vi "MoveRelate.vi"(8 "error in (no error)":errorcluster, 11 "DMC 3600 in":refnum<class "DMC 3600.lvclass">) -> (0 "error out":errorcluster, 3 "DMC 3600 out":refnum<class "DMC 3600.lvclass">)   [LabVIEW 2019, in "DMC 3600.lvclass"]
uses:
  DMC 3600.lvclass
  LLB/Commonly VI.lvlib
  LLB/DMC3600/LTDMC.lvlib
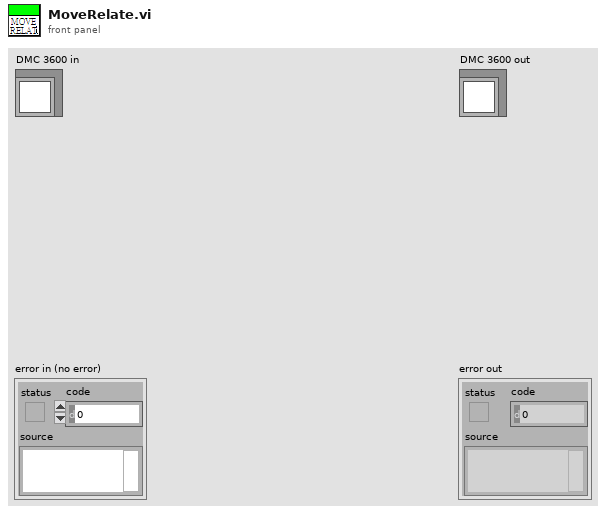
[diagram p1: front panel]
types:
  T1 = cluster{"AxisName":string, "Accel":dbl, "Deaccel":dbl, "Speed":dbl, "Sramp":dbl}[]
  T2 = cluster{"AxisName":string, "Accel":dbl, "Deaccel":dbl, "Speed":dbl, "Sramp":dbl}
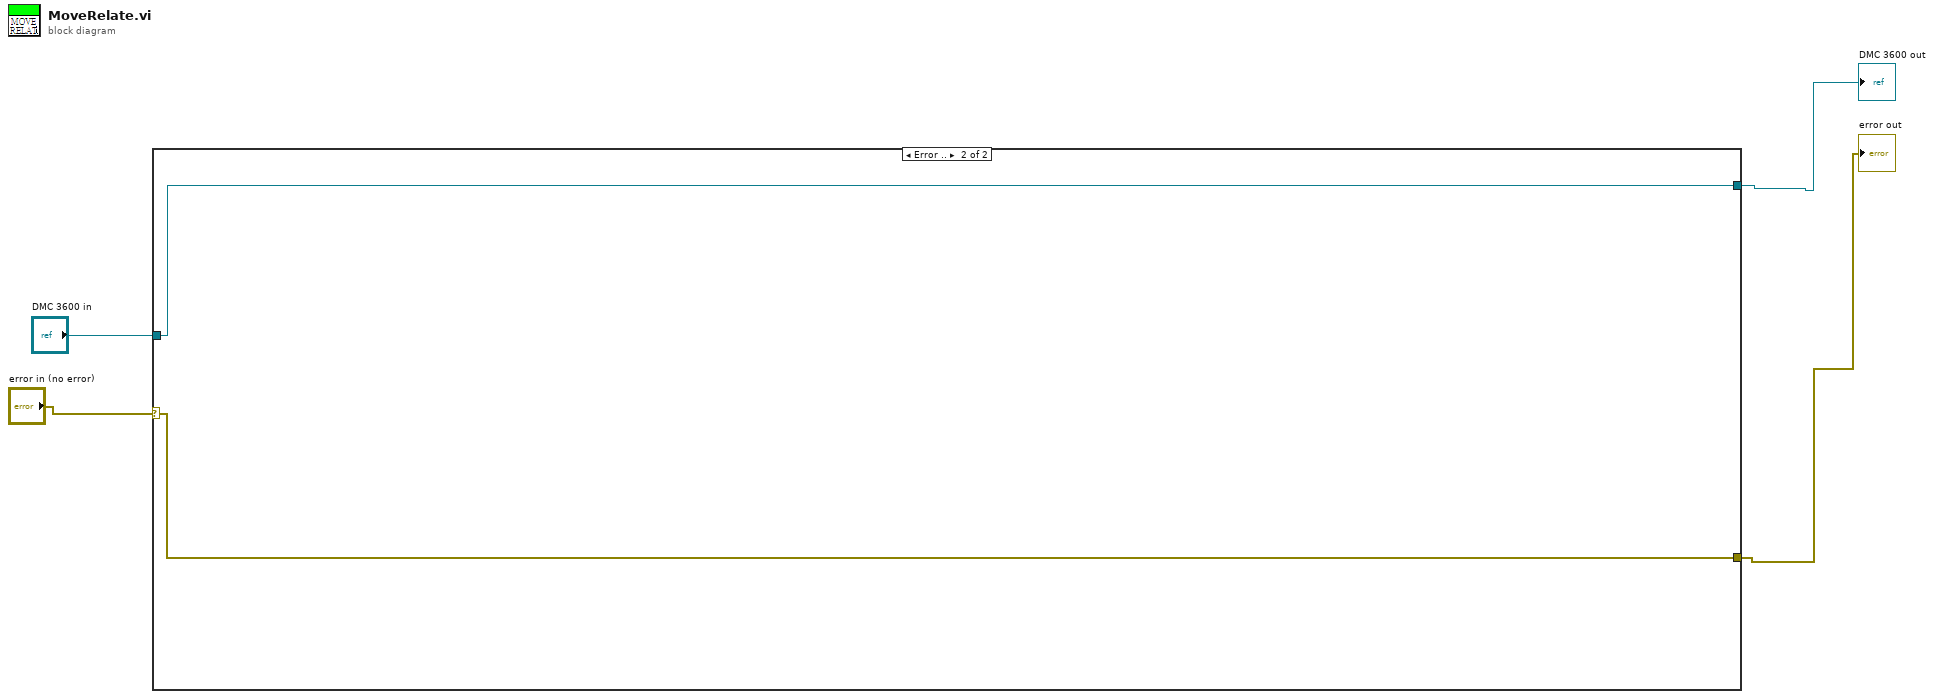
[diagram p0: block diagram]
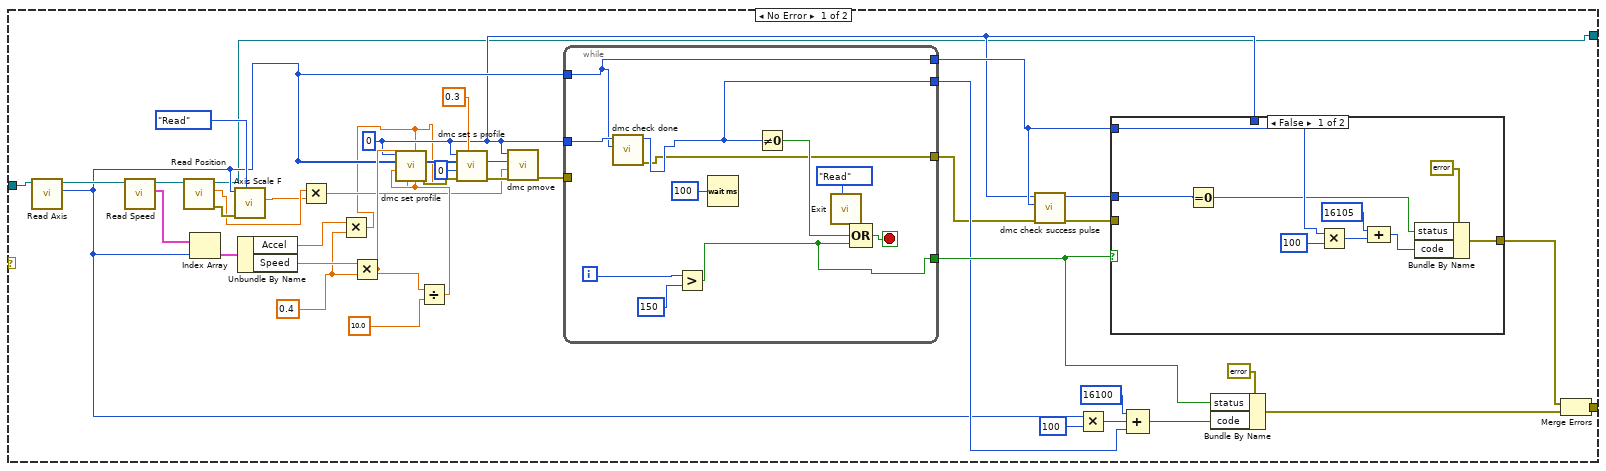
[diagram p2: hidden frame]
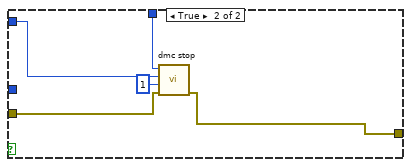
[diagram p3: hidden frame]
diagram:
  n1 = case shown="Error .." "error in (no error)" {
    selector: "error in (no error)" -> [_ w71]
    tunnel: [w10 w70] -> w4
    tunnel: [w9 w71] -> w3
    tunnel: "DMC 3600 in" -> [w8 w70]
    frame No Error {
      w6 = 0.4 ("y")
      w14 = u16 0 ("posi_mode")
      n2 = call-dynamic "Read Axis.vi"("AxisCard in"=w8) -> ("Axis"=w25:u32, "AxisCard out"=w43:refnum<class "DMC 3600.lvclass">)  [unwired: 8 in, 1 out]
      n3 = call-dynamic "Read Speed.vi"("AxisCard in"=w43) -> ("AxisSpeed"=w42:T1, "AxisCard out"=w33:refnum<class "DMC 3600.lvclass">)  [unwired: 8 in, 1 out]
      n4 = call-dynamic "Read Position.vi"("AxisCard in"=w33) -> ("error out"=w30:errorcluster, "Position"=w29:dbl, "AxisCard out"=w10:refnum<class "DMC 3600.lvclass">)  [unwired: 8 in]
      n5 = Index Array(array=w42, index=w25) -> (element=w41:T2)
      n6 = call "Axis Scale F.vi"("Enum"=enum16{"Initial", "Read"}."Read", "error In"=w30, "Axis"=w25) -> ("Scale"=w28:dbl)  [unwired: 7 in, 1 out]
      n7 = Unbundle By Name(w41) -> ("Accel"=w7:dbl, "Speed"=w31:dbl)
      n8 = Multiply(x=w29, y=w28) -> (x*y=w19:dbl)
      n9 = Multiply(x=w7, y=w6) -> (x*y=w5:dbl)
      n10 = Multiply(x=w31, y=w6) -> (x*y=w26:dbl)
      n11 = Divide(x=w26, y=10.0) -> (x/y=w24:dbl)
      n12 = call "dmc set profile.vi"("stop_vel"=w24, "Tdec"=w5, "Tacc"=w5, "Max_Vel"=w26, "Min_Vel"=w24, "axis"=w25, "CardNo"=w14) -> ("error out"=w23:errorcluster)  [unwired: 3 in, 1 out]
      n13 = call "dmc set s profile.vi"("s_para"=0.3, "error in (no error)"=w23, "s_mode"=u16 0, "axis"=w25, "CardNo"=w14) -> ("error out"=w22:errorcluster)  [unwired: 5 in, 1 out]
      n14 = call "dmc pmove.vi"("error in (no error)"=w22, "dist"=w19, "axis"=w25, "CardNo"=w14) -> ("error out"=w18:errorcluster)  [unwired: 6 in, 1 out]
      n15 = while {
        tunnel: w25 -> [w61]
        tunnel: [w61] -> w17
        tunnel: [w58] -> w35
        tunnel: [w60] -> w34
        tunnel: w18 -> [_]
        tunnel: w14 -> [w62]
        tunnel: [w59] -> w16
        i -> [w66]
        stop <- w67 stop-if-true
        n16 = call "dmc check done.vi"("axis"=w61, "CardNo"=w62) -> ("error out"=w59:errorcluster, "function return"=w60:i16)  [unwired: 8 in]
        n17 = Greater?(x=w66, y=u32 150) -> (0:w58:bool)
        n18 = Wait (ms)(milliseconds to wait=u32 100) -> ()  [unwired: 1 out]
        n19 = Not Equal To 0?(x=w60) -> (x != 0?=w63:bool)
        n20 = call "Exit.vi"("Enum"=enum16{"Initial", "Read", "Write"}."Read") -> ("ExitOut"=w65:bool)  [unwired: 10 in]
        n21 = Compound Arithmetic op=OR(w65, w63, w58) -> (w67:bool)
      }
      n22 = call "dmc check success pulse.vi"("error in (no error)"=w16, "axis"=w17, "CardNo"=w14) -> ("error out"=w13:errorcluster, "function return"=w12:i16)  [unwired: 7 in]
      n23 = Multiply(x=w25, y=u32 100) -> (x*y=w39:u32)
      n24 = case shown="False" w35 {
        tunnel: w17 -> [w48 w57]
        tunnel: w14 -> [_ w56]
        tunnel: w13 -> [_ w54]
        tunnel: w12 -> [w52 _]
        tunnel: [w44 w53] -> w11
        frame False {
          n25 = Equal To 0?(x=w52) -> (x = 0?=w45:bool)
          n26 = Multiply(x=w48, y=u32 100) -> (x*y=w50:u32)
          n27 = Compound Arithmetic op=ADD(16105, w50) -> (w46:u32)
          n28 = Bundle By Name(cluster=errorcluster {"status"=FALSE, "code"=0, "source"=""} ("error constant"), "status"=w45, "code"=w46) -> (w44:errorcluster)
        }
        frame True {
          n29 = call "dmc stop.vi"("error in (no error)"=w54, "stop_mode"=u16 1, "axis"=w57, "CardNo"=w56) -> ("error out"=w53:errorcluster)  [unwired: 6 in, 1 out]
        }
      }
      n30 = Compound Arithmetic op=ADD(16100, w39, w34) -> (w36:u32)
      n31 = Bundle By Name(cluster=errorcluster {"status"=FALSE, "code"=0, "source"=""} ("error constant"), "status"=w35, "code"=w36) -> (w15:errorcluster)
      n32 = Merge Errors(w11, w15) -> (w9:errorcluster)
    }
    frame Error {
    }
  }
  "error out" <- w3
  "DMC 3600 out" <- w4
